vi "Actor Core.vi"(8 "error in":errorcluster, 11 "TRExperimentsRaw in":refnum<class "Working Range.lvclass">) -> (0 "error out":errorcluster, 3 "Actor out":refnum<class "Actor.lvclass">)   [LabVIEW 2020, in "Forms.lvlib" / "Working Range.lvclass"]
doc: "The user interface for this panel.\n\n----\nPlease see the following web address for additional documentation and tutorial information:\nhttp://www.mooregoodideas.com/mgi-panel-manager/\n\nAuthor: Derek Trepanier\n\nCopyright (c) 2018, Moore Good Ideas, Inc.\n\nAll rights reserved.\n\nRedistribution and use in source and binary forms, with or without modification, are permitted provided that the following conditions are met:\n\n * Redistributions of source code must retain the above copyright notice, this list of conditions and the following disclaimer.\n * Redistributions in binary form must reproduce the above copyright notice, this list of conditions and the following disclaimer in the documentation and/or other materials provided with the distribution.\n * Neither the name of Moore Good Ideas, Inc. nor the names of its contributors may be used to endorse or promote products derived from this software without specific prior written permission.\n\nTHIS SOFTWARE IS PROVIDED BY THE COPYRIGHT HOLDERS AND CONTRIBUTORS \"AS IS\" AND ANY EXPRESS OR IMPLIED WARRANTIES, INCLUDING, BUT NOT LIMITED TO, THE IMPLIED WARRANTIES OF MERCHANTABILITY AND FITNESS FOR A PARTICULAR PURPOSE ARE DISCLAIMED. IN NO EVENT SHALL THE COPYRIGHT OWNER OR CONTRIBUTORS BE LIABLE FOR ANY DIRECT, INDIRECT, INCIDENTAL, SPECIAL, EXEMPLARY, OR CONSEQUENTIAL DAMAGES (INCLUDING, BUT NOT LIMITED TO, PROCUREMENT OF SUBSTITUTE GOODS OR SERVICES; LOSS OF USE, DATA, OR PROFITS; OR BUSINESS INTERRUPTION) HOWEVER CAUSED AND ON ANY THEORY OF LIABILITY, WHETHER IN CONTRACT, STRICT LIABILITY, OR TORT (INCLUDING NEGLIGENCE OR OTHERWISE) ARISING IN ANY WAY OUT OF THE USE OF THIS SOFTWARE, EVEN IF ADVISED OF THE POSSIBILITY OF SUCH DAMAGE."
uses:
  Working Range.lvclass
  C:/Users/User/Desktop/Raman Program/Database OOP/source/Forms AF/Form Controller/Panel Form Controller.lvclass
  <vilib>/ActorFramework/Actor/Actor.lvclass
  Samples/Samples.lvclass
  Form Controller/Panel Form Controller.lvclass/Panel Form Controller.ctl
  Database OOP/Column Libraries/Basic Fields/Field Configurations/Field Configuration Class/Field Configuration.lvclass
  C:/Users/User/Desktop/Raman Program/Database OOP/source/Database OOP/Column Libraries/Field Interfaces/Field Configuration Interface Class/Field Configuration.lvclass
  Open Form Button/Open Form Button.lvclass
  C:/Users/User/Desktop/Raman Program/Database OOP/source/Database OOP/Button Libraries/Button Interface Class/Button Interface.lvclass
  Database OOP/Column Libraries/Basic Field Constructors/Text Field.vi
  Database OOP/Column Libraries/Basic Field Constructors/FK Ring Field.vi
  Database OOP/Column Libraries/Basic Field Constructors/Numeric Field.vi
  Form Window/Form Window.lvclass
  Database OOP/Table Libraries/Basic Form/Basic Form.lvclass
  Database OOP/Column Libraries/Basic Field Constructors.lvlib
  Form Controller/Panel Form Controller.lvclass
panel:
  in  "Units":string
  in  "dy/dx":dbl
  in  "dz/dx":dbl
  in  "Z":dbl
  in  "Y Max":dbl
  in  "Y Min":dbl
  in  "X Max":dbl
  in  "X Min":dbl
  in  "Add Sample":bool
  in  "Display Name":string
  in  "Sample":u16(ring) items=["None"=1, "P"=2, "BSP"=3, "R"=4, "OC"=5, "undoped"=6, "A"=7, "S"=8]
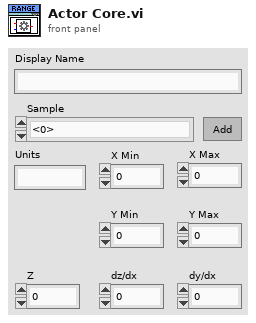
[diagram p1: front panel]
types:
  T1 = typedef "Panel Form Controller.lvlib/Builder Cluster.ctl" = cluster{"VI Ctrl Array":refnum<vi>[], "Form":refnum<class "Basic Form.lvclass">, "Open Form Button":refnum<class "Open Form Button.lvclass">}
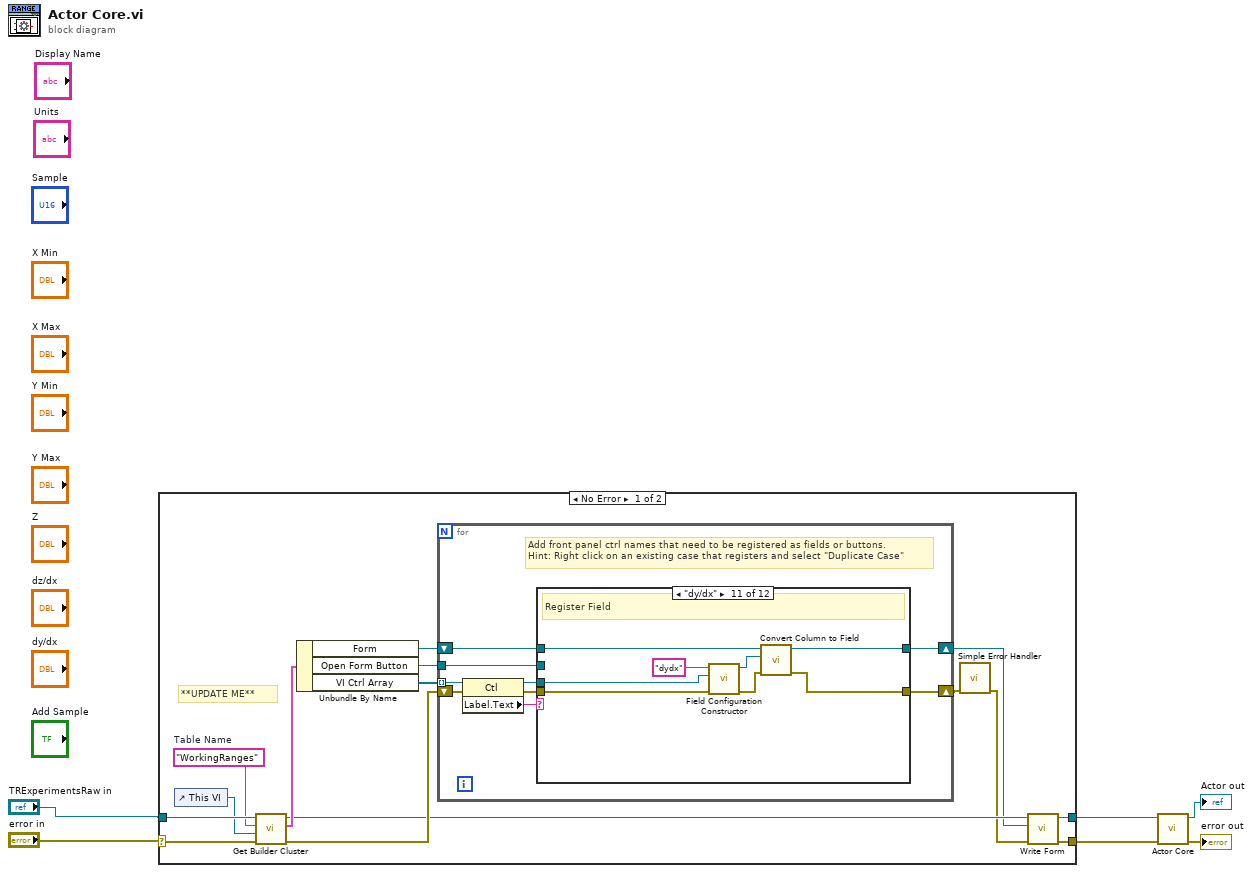
[diagram p0: block diagram]
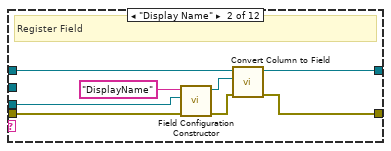
[diagram p3: hidden frame]
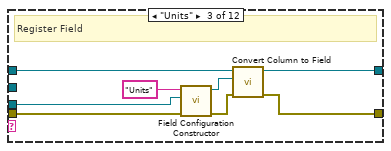
[diagram p4: hidden frame]
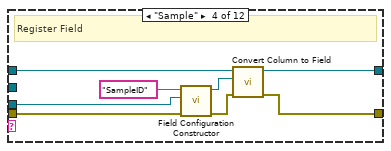
[diagram p5: hidden frame]
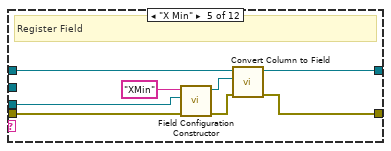
[diagram p6: hidden frame]
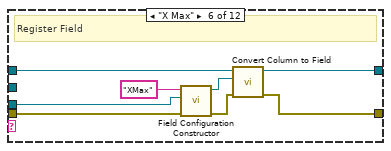
[diagram p7: hidden frame]
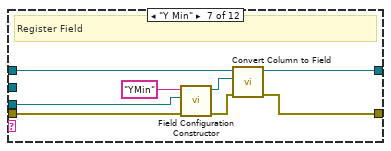
[diagram p8: hidden frame]
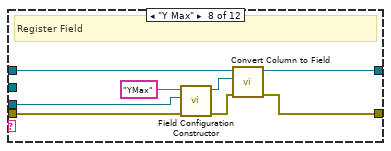
[diagram p9: hidden frame]
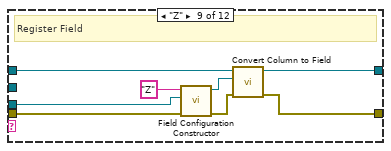
[diagram p10: hidden frame]
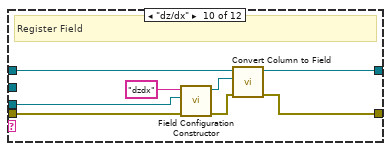
[diagram p11: hidden frame]
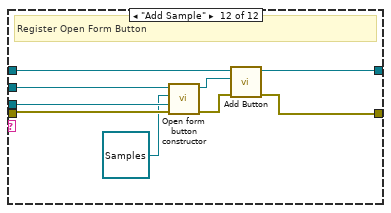
[diagram p12: hidden frame]
diagram:
  n1 = case shown="No Error" "error in" {
    selector: "error in" -> [w16 w123]
    tunnel: "TRExperimentsRaw in" -> [w20 w122]
    tunnel: [w9 w123] -> w1
    tunnel: [w10 w122] -> w2
    frame No Error {
      w7 = "WorkingRanges"  # Table Name
      # "**UPDATE ME**"
      n2 = control-ref of="This VI"() -> (w8:refnum<vi>)
      n3 = call "Get Builder Cluster.vi"("error in (no error)"=w16, "VI Refnum"=w8, "Table Name"=w7, "Panel Form Controller in"=w20) -> ("error out"=w18:errorcluster, "Builder Cluster"=w17:T1, "Panel Form Controller out"=w13:refnum<class "Working Range.lvclass">)  [unwired: 5 in]
      n4 = Unbundle By Name(w17) -> ("Form"=w19:refnum<class "Basic Form.lvclass">, "Open Form Button"=w14:refnum<class "Open Form Button.lvclass">, "VI Ctrl Array"=w15:refnum<vi>[])
      n5 = for {
        tunnel: w15 -> [w30] mode=indexing
        shift-right: [w23] -> w11
        shift-left: w19 -> [w24]
        shift-right: [w28] -> w21
        shift-left: w18 -> [w27]
        tunnel: w14 -> [w22]
        # "Add front panel ctrl names that need to be registered as fields or buttons.\nHint: Right click on an existing case that registers and select \"Duplicate Case\""
        n6 = property class="Ctl"(reference=w30, error in=w27) -> (reference out=w29:refnum<vi>, error out=w26:errorcluster, "Label.Text"=w25:string)
        n7 = case shown="\"dy/dx\"" w25 {
          tunnel: w29 -> [_ w35 w43 w51 w59 w67 w75 w83 w91 w99 w107 w115]
          tunnel: w24 -> [w32 w40 w48 w56 w64 w72 w80 w88 w96 w104 w112 w121]
          tunnel: [w32 w38 w46 w54 w62 w70 w78 w86 w94 w102 w110 w120] -> w23
          tunnel: [w31 w39 w47 w55 w63 w71 w79 w87 w95 w103 w111 w119] -> w28
          tunnel: w26 -> [w31 w34 w42 w50 w58 w66 w74 w82 w90 w98 w106 w114]
          tunnel: w22 -> [_ _ _ _ _ _ _ _ _ _ _ w116]
          frame "", Default {
            # "Not Registered"
          }
          frame "Display Name" {
            # "Register Field"
            n8 = call-poly "Field Configuration Constructor.vi"("error in"=w34, "Ctl Refnum"=w35, "Column Name"="DisplayName" ("Column")) -> ("error out"=w37:errorcluster, "Field Configuration"=w33:refnum<class "Field Configuration.lvclass">)  [unwired: 7 in]
            n9 = call "Convert Column to Field.vi"("error in (no error)"=w37, "Field Configuration"=w33, "Basic Form in"=w40) -> ("error out"=w39:errorcluster, "Basic Form out"=w38:refnum<class "Basic Form.lvclass">)  [unwired: 7 in]
          }
          frame "Units" {
            # "Register Field"
            n10 = call-poly "Field Configuration Constructor.vi"("error in"=w42, "Ctl Refnum"=w43, "Column Name"="Units" ("Column")) -> ("error out"=w45:errorcluster, "Field Configuration"=w41:refnum<class "Field Configuration.lvclass">)  [unwired: 7 in]
            n11 = call "Convert Column to Field.vi"("error in (no error)"=w45, "Field Configuration"=w41, "Basic Form in"=w48) -> ("error out"=w47:errorcluster, "Basic Form out"=w46:refnum<class "Basic Form.lvclass">)  [unwired: 7 in]
          }
          frame "Sample" {
            # "Register Field"
            n12 = call-poly "Field Configuration Constructor.vi"("error in"=w50, "Ctl Refnum"=w51, "Column Name"="SampleID" ("Column")) -> ("error out"=w53:errorcluster, "Field Configuration"=w49:refnum<class "Field Configuration.lvclass">)  [unwired: 7 in]
            n13 = call "Convert Column to Field.vi"("error in (no error)"=w53, "Field Configuration"=w49, "Basic Form in"=w56) -> ("error out"=w55:errorcluster, "Basic Form out"=w54:refnum<class "Basic Form.lvclass">)  [unwired: 7 in]
          }
          frame "X Min" {
            # "Register Field"
            n14 = call-poly "Field Configuration Constructor.vi"("error in"=w58, "Ctl Refnum"=w59, "Column Name"="XMin" ("Column")) -> ("error out"=w61:errorcluster, "Field Configuration"=w57:refnum<class "Field Configuration.lvclass">)  [unwired: 7 in]
            n15 = call "Convert Column to Field.vi"("error in (no error)"=w61, "Field Configuration"=w57, "Basic Form in"=w64) -> ("error out"=w63:errorcluster, "Basic Form out"=w62:refnum<class "Basic Form.lvclass">)  [unwired: 7 in]
          }
          frame "X Max" {
            # "Register Field"
            n16 = call-poly "Field Configuration Constructor.vi"("error in"=w66, "Ctl Refnum"=w67, "Column Name"="XMax" ("Column")) -> ("error out"=w69:errorcluster, "Field Configuration"=w65:refnum<class "Field Configuration.lvclass">)  [unwired: 7 in]
            n17 = call "Convert Column to Field.vi"("error in (no error)"=w69, "Field Configuration"=w65, "Basic Form in"=w72) -> ("error out"=w71:errorcluster, "Basic Form out"=w70:refnum<class "Basic Form.lvclass">)  [unwired: 7 in]
          }
          frame "Y Min" {
            # "Register Field"
            n18 = call-poly "Field Configuration Constructor.vi"("error in"=w74, "Ctl Refnum"=w75, "Column Name"="YMin" ("Column")) -> ("error out"=w77:errorcluster, "Field Configuration"=w73:refnum<class "Field Configuration.lvclass">)  [unwired: 7 in]
            n19 = call "Convert Column to Field.vi"("error in (no error)"=w77, "Field Configuration"=w73, "Basic Form in"=w80) -> ("error out"=w79:errorcluster, "Basic Form out"=w78:refnum<class "Basic Form.lvclass">)  [unwired: 7 in]
          }
          frame "Y Max" {
            # "Register Field"
            n20 = call-poly "Field Configuration Constructor.vi"("error in"=w82, "Ctl Refnum"=w83, "Column Name"="YMax" ("Column")) -> ("error out"=w85:errorcluster, "Field Configuration"=w81:refnum<class "Field Configuration.lvclass">)  [unwired: 7 in]
            n21 = call "Convert Column to Field.vi"("error in (no error)"=w85, "Field Configuration"=w81, "Basic Form in"=w88) -> ("error out"=w87:errorcluster, "Basic Form out"=w86:refnum<class "Basic Form.lvclass">)  [unwired: 7 in]
          }
          frame "Z" {
            # "Register Field"
            n22 = call-poly "Field Configuration Constructor.vi"("error in"=w90, "Ctl Refnum"=w91, "Column Name"="Z" ("Column")) -> ("error out"=w93:errorcluster, "Field Configuration"=w89:refnum<class "Field Configuration.lvclass">)  [unwired: 7 in]
            n23 = call "Convert Column to Field.vi"("error in (no error)"=w93, "Field Configuration"=w89, "Basic Form in"=w96) -> ("error out"=w95:errorcluster, "Basic Form out"=w94:refnum<class "Basic Form.lvclass">)  [unwired: 7 in]
          }
          frame "dz/dx" {
            # "Register Field"
            n24 = call-poly "Field Configuration Constructor.vi"("error in"=w98, "Ctl Refnum"=w99, "Column Name"="dzdx" ("Column")) -> ("error out"=w101:errorcluster, "Field Configuration"=w97:refnum<class "Field Configuration.lvclass">)  [unwired: 7 in]
            n25 = call "Convert Column to Field.vi"("error in (no error)"=w101, "Field Configuration"=w97, "Basic Form in"=w104) -> ("error out"=w103:errorcluster, "Basic Form out"=w102:refnum<class "Basic Form.lvclass">)  [unwired: 7 in]
          }
          frame "dy/dx" {
            # "Register Field"
            n26 = call-poly "Field Configuration Constructor.vi"("error in"=w106, "Ctl Refnum"=w107, "Column Name"="dydx" ("Column")) -> ("error out"=w109:errorcluster, "Field Configuration"=w105:refnum<class "Field Configuration.lvclass">)  [unwired: 7 in]
            n27 = call "Convert Column to Field.vi"("error in (no error)"=w109, "Field Configuration"=w105, "Basic Form in"=w112) -> ("error out"=w111:errorcluster, "Basic Form out"=w110:refnum<class "Basic Form.lvclass">)  [unwired: 7 in]
          }
          frame "Add Sample" {
            # "Register Open Form Button"
            n28 = call "Open form button constructor.vi"("error in (no error)"=w114, "Ctl Refnum"=w115, "Panel Form"=refnum<class "Samples.lvclass"> refnum ("Forms.lvlib:Samples.lvclass"), "Open Form Button in"=w116) -> ("error out"=w117:errorcluster, "Open Form Button out"=w118:refnum<class "Open Form Button.lvclass">)  [unwired: 6 in]
            n29 = call "Add Button.vi"("error in (no error)"=w117, "Button"=w118, "Basic Form in"=w121) -> ("error out"=w119:errorcluster, "Basic Form out"=w120:refnum<class "Basic Form.lvclass">)  [unwired: 7 in]
          }
        }
      }
      n30 = call <vilib>:"Simple Error Handler.vi"("error in (no error)"=w21) -> ("error out"=w12:errorcluster)  [unwired: 4 in, 4 out]
      n31 = call "Write Form.vi"("error in (no error)"=w12, "Form.lvlib:Basic Form.lvclass"=w11, "Panel Form Controller in"=w13) -> ("error out"=w9:errorcluster, "Panel Form Controller out"=w10:refnum<class "Working Range.lvclass">)  [unwired: 7 in]
    }
    frame Error {
    }
  }
  n32 = call-parent "Actor Core.vi"("error in"=w1, "Form Window in"=w2) -> ("error out"=→"error out":errorcluster, "Actor out"=→"Actor out":refnum<class "Actor.lvclass">)  [unwired: 8 in]
